vi "Receive Message.vi"(6 "priority":i32, 10 "Common in":refnum<class "Common.lvclass">, 11 "Message in":refnum<class "Message.lvclass">) -> (0 "error out":errorcluster, 2 "Actor out":refnum<class "Actor.lvclass">)   [LabVIEW 2021, in "Common.lvlib" / "Common.lvclass"]
doc: "This VI should be overriden ONLY if you are creating a proxy actor for remote transmission. If you are, override this VI to transmit the received message to a new destination, maintaining the given priority."
uses:
  <vilib>/ActorFramework/Message/Message.lvclass
  <vilib>/ActorFramework/Actor/Actor.lvclass
  Common.lvclass
  Common.lvclass/Common.ctl
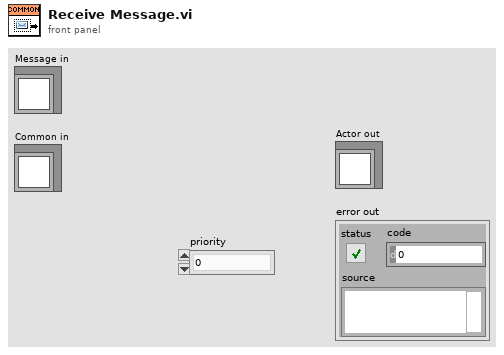
[diagram p1: front panel]
types:
  T1 = cluster{"message":string, "payload":string, "timestamp":timestamp}
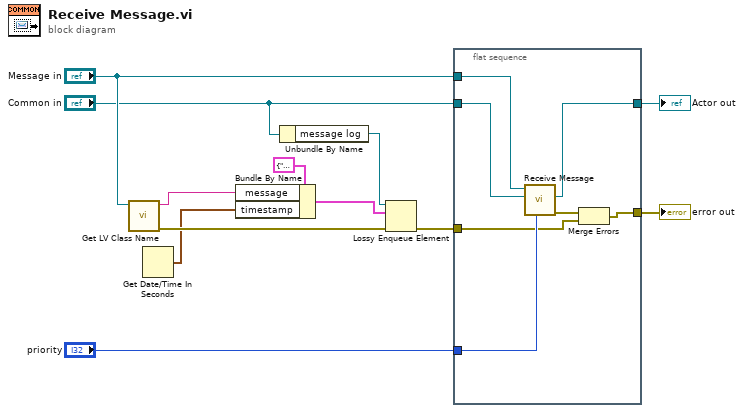
[diagram p0: block diagram]
diagram:
  n1 = call <vilib>:"Get LV Class Name.vi"("object"="Message in") -> ("error out"=w7:errorcluster, "class name"=w4:string)  [unwired: 9 in]
  n2 = Get Date/Time In Seconds() -> (seconds since 1Jan1904=w1:timestamp)
  n3 = Bundle By Name(cluster=T1 {"message"="", "payload"="", "timestamp"=timestamp(0 s since 1904-01-01)}, "message"=w4, "timestamp"=w1) -> (w3:T1)
  n4 = Unbundle By Name("Common in") -> ("message log"=w5:refnum<queue>)
  n5 = Lossy Enqueue Element(queue=w5, element=w3, error in (no error)=w7) -> (error out=w6:errorcluster)  [unwired: 3 out]
  n6 = flat-sequence {
    tunnel: [w18] -> w12
    tunnel: "priority" -> [w17]
    tunnel: "Common in" -> [w16]
    tunnel: "Message in" -> [w15]
    tunnel: [w14] -> w9
    tunnel: w6 -> [w13]
    frame #0 {
      n7 = call-parent "Receive Message.vi"("priority"=w17, "Actor in"=w16, "Message in"=w15) -> ("error out"=w19:errorcluster, "Actor out"=w18:refnum<class "Actor.lvclass">)  [unwired: 7 in]
      n8 = Merge Errors(w19, w13) -> (w14:errorcluster)
    }
  }
  "error out" <- w9
  "Actor out" <- w12
